vi "Get Module Main VI Information.vi"(8 "error in":errorcluster) -> (0 "error out":errorcluster, 1 "Execution State":T1(ring), 2 "Is Module Running?":bool, 3 "Module Main VI":refnum<vi>)   [LabVIEW 2020, in "Settings Editor.lvlib"]
doc: "Return information about the module main VI, including its VI reference, its execution state enum, and a Boolean value indicating whether or not it is running.\n_____\nBased on DQMH Project Template 4.0.0.47.\n_____\nBased on DQMH Project Template 7.0.1.1316."
uses:
  Settings Editor.lvlib
  Main.vi
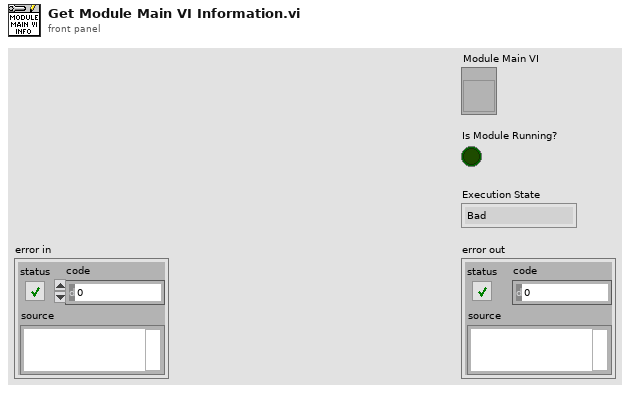
[diagram p1: front panel]
types:
  T1 = enum32{"Bad", "Idle", "Run top level", "Running"}
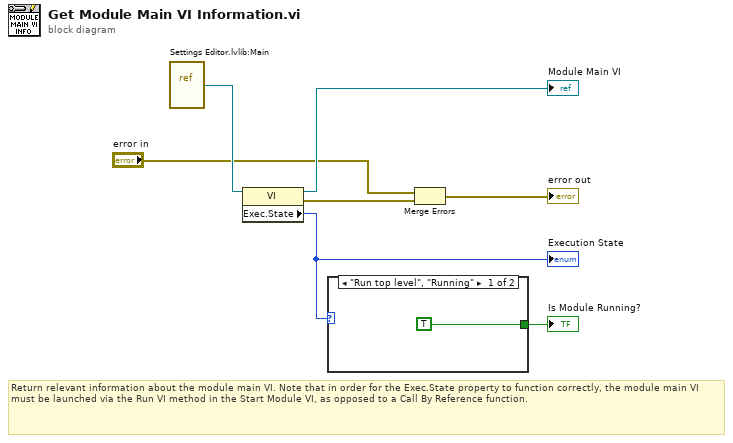
[diagram p0: block diagram]
diagram:
  # "Return relevant information about the module main VI. Note that in order for the Exec.State property to function correctly, the module main VI must be launched via the Run VI method in the Start Module VI, as opposed to a Call By Reference function."
  n1 = vi-ref "Settings Editor.lvlib:Main.vi"() -> (w5:refnum<vi>)
  n2 = property on="Property Node" class="VI"(reference=w5) -> (reference out=→"Module Main VI":refnum<vi>, error out=w6:errorcluster, "Exec.State"=w4:T1)  [unwired: 1 in]
  "Execution State" <- w4
  n3 = case shown="\"Run top level\", \"Running\"" w4 {
    tunnel: [TRUE _] -> w3
    frame "Run top level", "Running" {
    }
    frame "Bad", "Idle" {
    }
  }
  "Is Module Running?" <- w3
  n4 = Merge Errors("error in", w6) -> (→"error out":errorcluster)
